vi "parse_image.vi"(4 "error in":errorcluster, 7 "msg in":string) -> (0 "error out":errorcluster, 1 "Image Out":T1 {"Dialogs" format="%.0b"}, 2 "ROS Image":T2, 3 "msg out":string)   [LabVIEW 2010]
uses:
  <userlib>/ImageProcessing/QTLIB_2595_LV86/QT_Image.ctl
  <userlib>/ROSforLV/ROS/parsing/std_msgs/subs/parse_u32_scalar.vi
  <userlib>/ROSforLV/ROS/parsing/std_msgs/subs/parse_string_scalar.vi
  <userlib>/ROSforLV/ROS/parsing/std_msgs/subs/parse_u8_scalar.vi
  <userlib>/ROSforLV/ROS/parsing/std_msgs/subs/parse_u8_array.vi
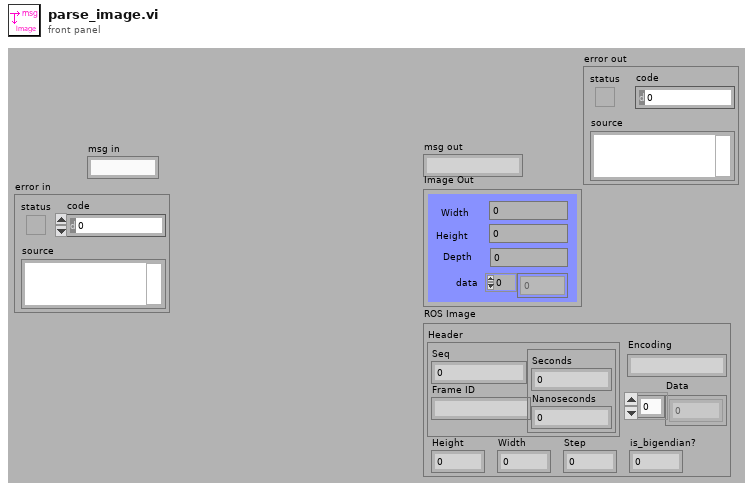
[diagram p1: front panel]
types:
  T1 = typedef "QT_Image.ctl" = cluster{"Width":i32, "Height":i32, "Depth":i32, "data":u8[], "Compressed data":u8[], "Color table":u32[], "Duration":i32, "Options":i32, "Timestamp":i32, "ID":i32, "Reserved":i32, "Dialogs":u32}
  T2 = cluster{"Header":cluster{"Seq":u32, "Frame ID":string, cluster{"Seconds":i32, "Nanoseconds":i32}}, "Height":u32, "Width":u32, "is_bigendian?":u8, "Step":u32, "Data":u8[], "Encoding":string}
  T3 = cluster{"Seq":u32, "Frame ID":string, "Timestamp":cluster{"Seconds":i32, "Nanoseconds":i32}}
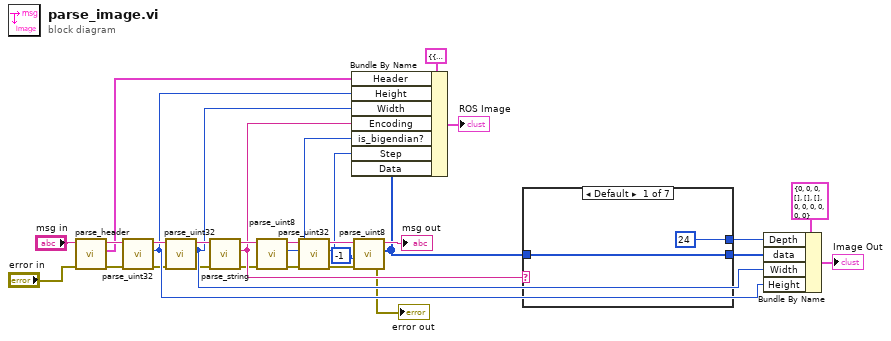
[diagram p0: block diagram]
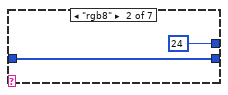
[diagram p2: hidden frame]
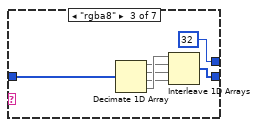
[diagram p3: hidden frame]
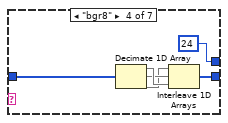
[diagram p4: hidden frame]
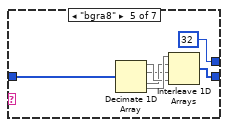
[diagram p5: hidden frame]
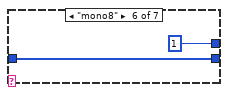
[diagram p6: hidden frame]
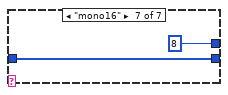
[diagram p7: hidden frame]
diagram:
  n1 = call <userlib>:"parse_header.vi"("error in"="error in", "msg in"="msg in") -> ("error out"=w3:errorcluster, "Header"=w22:T3, "msg out"=w30:string)  [unwired: 3 in]
  n2 = call-poly <userlib>:"parse_uint32.vi"("error in"=w3, "msg in"=w30) -> ("error out"=w4:errorcluster, "number"=w10:u32, "msg out"=w29:string)  [unwired: 3 in]
  n3 = call-poly <userlib>:"parse_uint32.vi"("error in"=w4, "msg in"=w29) -> ("error out"=w5:errorcluster, "number"=w11:u32, "msg out"=w28:string)  [unwired: 3 in]
  n4 = call-poly <userlib>:"parse_string.vi"("error in"=w5, "msg in"=w28) -> ("error out"=w6:errorcluster, "string"=w14:string, "msg out"=w27:string)  [unwired: 3 in]
  n5 = call-poly <userlib>:"parse_uint8.vi"("error in"=w6, "msg in"=w27) -> ("error out"=w7:errorcluster, "number"=w21:u8, "msg out"=w26:string)  [unwired: 3 in]
  n6 = call-poly <userlib>:"parse_uint32.vi"("error in"=w7, "msg in"=w26) -> ("error out"=w8:errorcluster, "number"=w20:u32, "msg out"=w25:string)  [unwired: 3 in]
  n7 = call-poly <userlib>:"parse_uint8.vi"("error in"=w8, "Array Size"=-1, "msg in"=w25) -> ("error out"=→"error out":errorcluster, "number"=w15:u8[], "msg out"=→"msg out":string)  [unwired: 2 in]
  n8 = Bundle By Name(cluster=T2 {"Header"={"Seq"=0, "Frame ID"="", {"Seconds"=0, "Nanoseconds"=0}}, "Height"=0, "Width"=0, "is_bigendian?"=0, "Step"=0, "Data"=[], "Encoding"=""} ("ROS Image"), "Header"=w22, "Height"=w10, "Width"=w11, "Encoding"=w14, "is_bigendian?"=w21, "Step"=w20, "Data"=w15) -> (→"ROS Image":T2)
  n9 = case shown="Default" w14 {
    tunnel: w15 -> [w32 w34 w40 w47 w54 w56 w58]
    tunnel: [w32 w34 w39 w46 w53 w56 w58] -> w12
    tunnel: [24 ("Depth") 24 ("Depth") 32 ("Depth") 24 ("Depth") 32 ("Depth") 1 ("Depth") 8 ("Depth")] -> w13
    frame Default {
    }
    frame "rgb8" {
    }
    frame "rgba8" {
      n10 = Decimate 1D Array(w40) -> (w37:u8[], w36:u8[], w35:u8[], w38:u8[])
      n11 = Interleave 1D Arrays(w38, w37, w36, w35) -> (w39:u8[])
    }
    frame "bgr8" {
      n12 = Decimate 1D Array(w47) -> (w45:u8[], w44:u8[], w43:u8[])
      n13 = Interleave 1D Arrays(w43, w44, w45) -> (w46:u8[])
    }
    frame "bgra8" {
      n14 = Decimate 1D Array(w54) -> (w50:u8[], w48:u8[], w49:u8[], w51:u8[])
      n15 = Interleave 1D Arrays(w51, w49, w48, w50) -> (w53:u8[])
    }
    frame "mono8" {
    }
    frame "mono16" {
    }
  }
  n16 = Bundle By Name(cluster=T1 {"Width"=0, "Height"=0, "Depth"=0, "data"=[], "Compressed data"=[], "Color table"=[], "Duration"=0, "Options"=0, "Timestamp"=0, "ID"=0, "Reserved"=0, "Dialogs"=0} ("Image Out"), "Depth"=w13, "data"=w12, "Width"=w11, "Height"=w10) -> (→"Image Out":T1)
